vi "Draw Intersections On XY Graph.vi"(11 "CombinedAnchorArray In":refnum<class "Anchor.lvclass">[](array[class])) -> (3 "XY Graph Out":cluster{"x":dbl[], "y":dbl[]}[](graph))   [LabVIEW 2014, in "Anchor.lvclass"]
doc: "This VI draws all the intersection circles on a XY Graph\naccording to its input"
uses:
  Anchor/Anchor.lvclass
  Anchor/Anchor.lvclass/Anchor.ctl
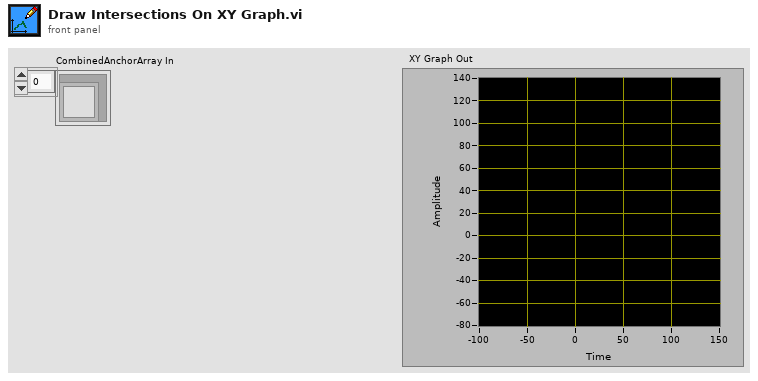
[diagram p1: front panel]
types:
  T1 = cluster{"Tag.lvclass":refnum<class "Tag.lvclass">, "Distance":dbl}[]
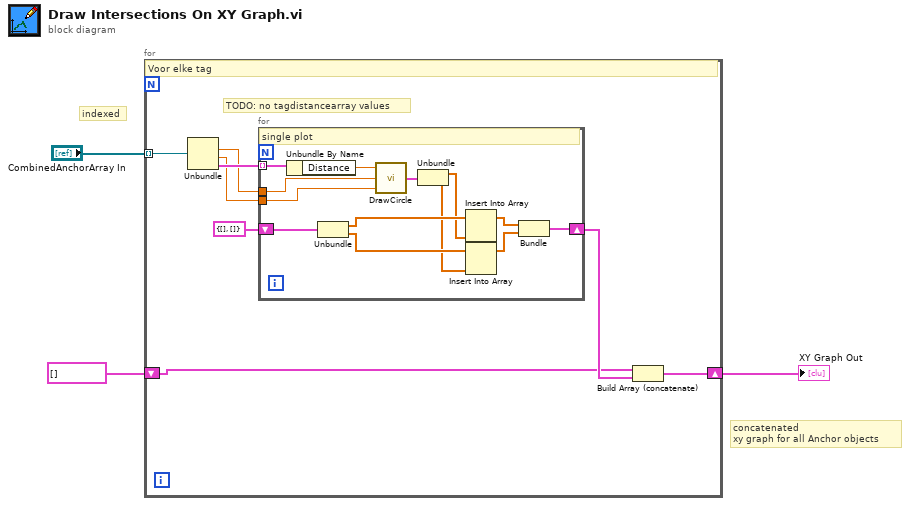
[diagram p0: block diagram]
diagram:
  # "concatenated\nxy graph for all Anchor objects"
  # "indexed"
  n1 = for {
    tunnel: "CombinedAnchorArray In" -> [w11] mode=indexing
    shift-right: [w4] -> w1
    shift-left: cluster{"x":dbl[], "y":dbl[]}[] [] -> [w5]
    # "TODO: no tagdistancearray values"
    # "Voor elke tag"
    n2 = Unbundle(w11) -> (w9:dbl, w8:dbl, w10:T1)  [unwired: 1 out]
    n3 = for {
      tunnel: w10 -> [w24] mode=indexing
      tunnel: w9 -> [w22]
      tunnel: w8 -> [w21]
      shift-right: [w12] -> w6
      shift-left: cluster{dbl[], dbl[]} {[], []} ("XY Graph 2") -> [w19]
      # "single plot"
      n4 = Unbundle By Name(w24) -> ("Distance"=w23:dbl)
      n5 = Unbundle(w19) -> (w18:dbl[], w17:dbl[])
      n6 = call "DrawCircle.vi"("y"=w21, "x"=w22, "r"=w23) -> ("XY Graph"=w20:cluster{dbl[], dbl[]})
      n7 = Unbundle(w20) -> (w16:dbl[], w15:dbl[])
      n8 = Insert Into Array(array=w18, new element=w16) -> (w14:dbl[])  [unwired: 1 in]
      n9 = Insert Into Array(array=w17, new element=w15) -> (w13:dbl[])  [unwired: 1 in]
      n10 = Bundle(w14, w13) -> (w12:cluster{dbl[], dbl[]})  [unwired: 1 in]
    }
    n11 = Build Array (concatenate)(w5, w6) -> (w4:cluster{"x":dbl[], "y":dbl[]}[])
  }
  "XY Graph Out" <- w1
